vi "ADIS16448 Loop Post Scale.vi"(6 "TimePeriod":dbl, 8 "Reset":bool, 9 "Data In":dbl[](array[numeric]), 10 "Offsets":dbl[](array[numeric]), 11 "Scaled Data In":dbl[](array[numeric])) -> (2 "Reset Out":bool, 3 "Data Out":dbl[](array[numeric]))   [LabVIEW 2019]
uses:
  ADIS16448 Globals.vi
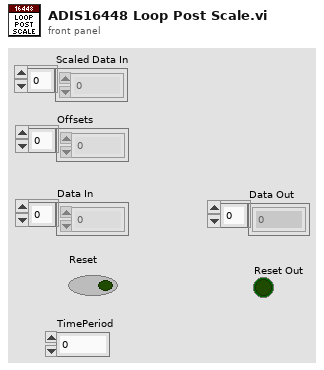
[diagram p1: front panel]
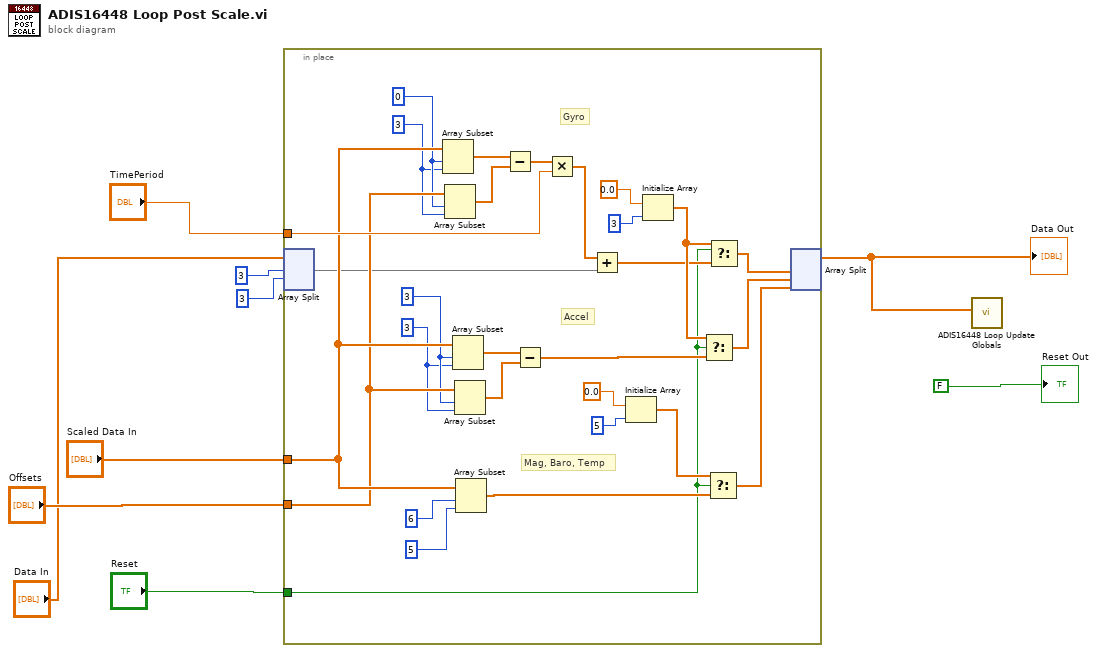
[diagram p0: block diagram]
diagram:
  n1 = in-place {
    in-place-border: "TimePeriod" -> [w38]
    in-place-border: "Reset" -> [w10]
    in-place-border: "Scaled Data In" -> [w37]
    in-place-border: "Offsets" -> [w36]
    w25 = 3 ("length")
    w26 = 3 ("index")
    w29 = 3 ("length")
    w30 = 0 ("index")
    # "Mag, Baro, Temp"
    # "Accel"
    # "Gyro"
    n2 = in-place-split #1("Data In", 3, 3) -> (w35:dbl[])  [unwired: 2 out]
    n3 = Array Subset(array=w37, index=w30, length=w29) -> (w32:dbl[])
    n4 = Array Subset(array=w36, index=w30, length=w29) -> (w31:dbl[])
    n5 = Array Subset(array=w37, index=w26, length=w25) -> (w28:dbl[])
    n6 = Array Subset(array=w36, index=w26, length=w25) -> (w27:dbl[])
    n7 = Array Subset(array=w37, index=6, length=5) -> (w13:dbl[])
    n8 = Subtract(x=w32, y=w31) -> (x-y=w34:dbl[])
    n9 = Subtract(x=w28, y=w27) -> (x-y=w15:dbl[])
    n10 = Multiply(x=w34, y=w38) -> (x*y=w33:dbl[])
    n11 = Add(x=w33, y=w35) -> (x+y=w17:dbl[])
    n12 = Initialize Array(0.0 ("element"), 5 ("dimension size")) -> (w12:dbl[])
    n13 = Initialize Array(0.0 ("element"), 3 ("dimension size")) -> (w18:dbl[])
    n14 = Select(t=w18, s=w10, f=w15) -> (s? t:f=w14:dbl[])
    n15 = Select(t=w12, s=w10, f=w13) -> (s? t:f=w11:dbl[])
    n16 = Select(t=w18, s=w10, f=w17) -> (s? t:f=w16:dbl[])
    n17 = in-place-split #1(w16, w14, w11) -> (w1:dbl[])  [unwired: 2 out]
  }
  "Data Out" <- w1
  n18 = call "ADIS16448 Loop Update Globals.vi"("Data In"=w1) -> ()  [unwired: 10 in, 1 out]
  "Reset Out" <- FALSE ("Reset")
